vi "Close.vi"(8 "error in (no error)":errorcluster, 11 "Controlador in":refnum<class "Controlador.lvclass">) -> (0 "error out":errorcluster, 3 "Controlador out":refnum<class "Controlador.lvclass">)   [LabVIEW 2018, in "Controlador.lvclass"]
uses:
  Controlador.lvclass
  Controlador.lvclass/Controlador.ctl
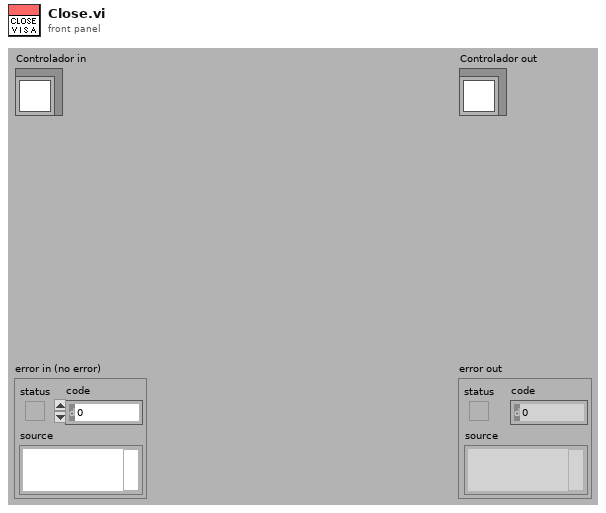
[diagram p1: front panel]
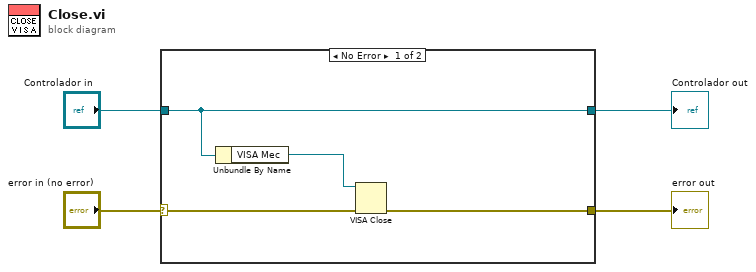
[diagram p0: block diagram]
diagram:
  n1 = case shown="No Error" "error in (no error)" {
    selector: "error in (no error)" -> [w6 w9]
    tunnel: "Controlador in" -> [w8 w10]
    tunnel: [w8 w10] -> w1
    tunnel: [w5 w9] -> w2
    frame No Error {
      n2 = Unbundle By Name(w8) -> ("VISA Mec"=w7:refnum<visa-resource-name>)
      n3 = VISA Close(VISA resource name=w7, error in (no error)=w6) -> (error out=w5:errorcluster)
    }
    frame Error {
    }
  }
  "error out" <- w2
  "Controlador out" <- w1
